vi "Upsample data.vi"(7 "factor":dbl, 11 "data":dbl[](array[numeric])) -> (3 "upsampled data":dbl[](array[numeric]))   [LabVIEW 2012]
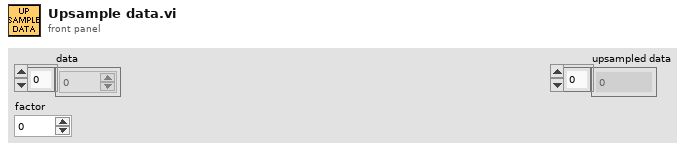
[diagram p1: front panel]
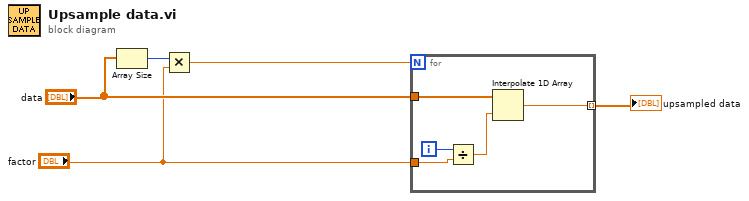
[diagram p0: block diagram]
diagram:
  n1 = Array Size(array="data") -> (size(s)=w5:i32)
  n2 = Multiply(x=w5, y="factor") -> (x*y=w4:dbl)
  n3 = for {
    N: w4 -> [_]
    tunnel: "factor" -> [w9]
    tunnel: "data" -> [w8]
    tunnel: [w6] -> w3 mode=indexing
    i -> [w10]
    n4 = Divide(x=w10, y=w9) -> (x/y=w7:dbl)
    n5 = Interpolate 1D Array(1:w7, 2:w8) -> (0:w6:dbl)
  }
  "upsampled data" <- w3
